vi "SteppperMotorTest.vi"() -> ()   [LabVIEW 2019]
uses:
  WSCbot_V3_Toolkit.lvlibp/WSCBOTV3_Toolkit/IO/LowLevel/PulseCounter.ctl
  <vilib>/Platform/TimedLoop/XDataNode/timing_clust.ctl
  <vilib>/Platform/TimedLoop/XDataNode/nitl_modes.ctl
  <vilib>/Platform/TimedLoop/XDataNode/wakeup.ctl
  WSCbot_V3_Toolkit.lvlibp/WSCBOTV3_Toolkit/IO/LowLevel/IO_Chanel_DIO.ctl
  <vilib>/platform/TimedLoop/XDataNode/XDataNode.xnode
  WSCbot_V3_Toolkit.lvlibp
  <vilib>/Platform/TimedLoop/XDataNode/XDNodeRunTimeDep.lvlib
  WSCbot_V3_Toolkit.lvlibp/WSCBOTV3_Toolkit/MotorControl/LowLevel/ZaxisSlideSet.vi
panel:
  in  "PulseCounterChanel":T1
  in  "Refresh Button":bool
  out "PulseCount":i32
  in  "Stop":bool
  in  "positive/nagative":bool
  in  "Stop Button":bool
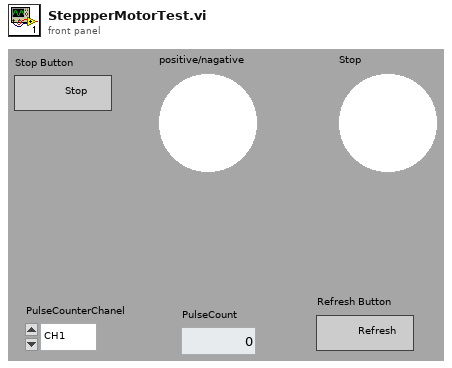
[diagram p1: front panel]
types:
  T1 = typedef "WSCbot_V3_Toolkit.lvlibp/PulseCounter.ctl" = enum16{"CH1", "CH2", "CH3", "CH4", "CH5"}
  T2 = typedef "XDNodeRunTimeDep.lvlib/timing_clust.ctl" = cluster{"Expected End [f-1]":u64, "Actual End [f-1]":u64, "Finished Late? [f-1]":bool, "Expected End [i-1]":u64, "Actual End [i-1]":u64, "Finished Late? [i-1]":bool, "Expected Start [i]":u64, "Actual Start [i]":u64, "Expected Start [f]":u64, "Actual Start [f]":u64, "Source Name":string, "Structure Name":string, "Period":i64, "Deadline":i64, "Offset":i64, "Start":i64, "Priority":i32, "Timeout":i32, "Mode":T3, "Wakeup Reason":T4, "Error":errorcluster, "Source Type":string, "Secondary Source Type":string, "Global End Time":u64, "Global Start Time":u64, "Frame Duration":u64, "Iteration Duration":u64, "Assigned CPU":i32, "I/O Scan Engine Mode":u32}
  T3 = typedef "XDNodeRunTimeDep.lvlib/nitl_modes.ctl" = enum32{"No Change", "Process missed periods, maintain original phase", "Discard missed periods, maintain original phase", "Process missed periods, ignore original phase", "Discard missed periods, ignore original phase"}
  T4 = typedef "XDNodeRunTimeDep.lvlib/wakeup.ctl" = enum32{"Normal", "Aborted", "Asynchronous wakeup", "Timing source error", "Timed loop error", "Timeout"}
  T5 = typedef "WSCbot_V3_Toolkit.lvlibp/IO_Chanel_DIO.ctl" = enum16{"A/DIO9", "A/DIO10", "C/DIO0", "C/DIO1", "C/DIO2", "C/DIO3", "C/DIO4", "C/DIO5", "C/DIO6"}
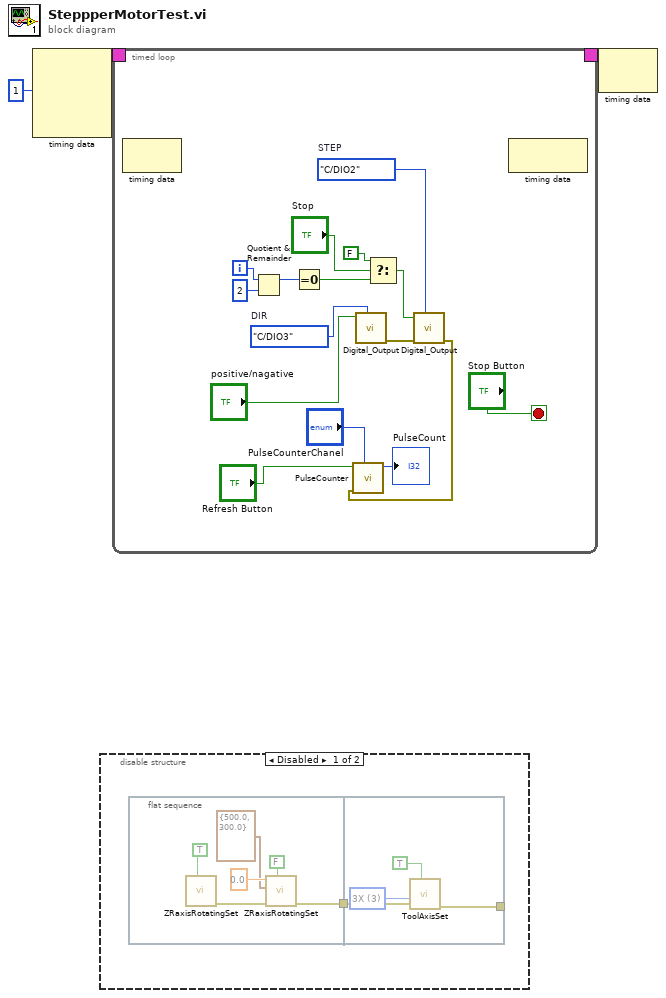
[diagram p0: block diagram]
diagram:
  n1 = node-c288(i64 1 ("Period")) -> (w3:T2)  [unwired: 3 in]
  n2 = disable-structure shown="Disabled" {
    frame Disabled {
      n3 = flat-sequence {
        tunnel: [w8] -> w4
        tunnel: w4 -> [w14]
        tunnel: [w11] -> _
        frame #0 {
          n4 = call "ZRaxisRotatingSet.vi"("Reset"=TRUE) -> ("error out"=w9:errorcluster)  [unwired: 9 in, 1 out]
          n5 = call "ZRaxisRotatingSet.vi"("Reset"=FALSE, "error in"=w9, "Velocity(deg/s)&ACC(deg/ss)"=cluster{"Velocity(cm/s)":dbl, "ACC(cm/ss)":dbl} {"Velocity(cm/s)"=500.0, "ACC(cm/ss)"=300.0}, "TargetHight(deg)"=0.0) -> ("error out"=w8:errorcluster)  [unwired: 6 in, 1 out]
        }
        frame #1 {
          w12 = u16 3 items=["0X", "1X", "2X", "3X"] ("findHomeVel (times)")
          n6 = call-poly "ToolAxisSet.vi"("Reset"=TRUE, "error in"=w14, "findHomeVel (times)"=w12) -> ("error out"=w11:errorcluster)  [unwired: 7 in, 1 out]
        }
      }
    }
    frame Enabled {
    }
  }
  n7 = timed-loop {
    timing: w3 -> [_]
    timing-out: [_] -> w2
    i -> [w22]
    stop <- "Stop Button" stop-if-true
    w29 = IO_Chanel_DIO."C/DIO3"  # DIR
    w30 = IO_Chanel_DIO."C/DIO2"  # STEP
    n8 = node-c288() -> ()  [unwired: 1 in, 1 out]
    n9 = Quotient & Remainder(x=w22, y=2) -> (x-y*floor(x/y)=w20:i32)  [unwired: 1 out]
    n10 = Equal To 0?(x=w20) -> (x = 0?=w19:bool)
    n11 = call "Digital_Output.vi"("IO_Chanel"=w29, "False/True"="positive/nagative") -> ("error out"=w23:errorcluster)  [unwired: 9 in]
    n12 = Select(t=FALSE ("s"), s="Stop", f=w19) -> (s? t:f=w25:bool)
    n13 = call "Digital_Output.vi"("IO_Chanel"=w30, "error in"=w23, "False/True"=w25) -> ("error out"=w16:errorcluster)  [unwired: 8 in]
    n14 = call "PulseCounter.vi"("PulseCounterChanel"="PulseCounterChanel", "error in"=w16, "Reset"="Refresh Button") -> ("PulseCount"=→"PulseCount":i32)  [unwired: 7 in, 1 out]
    n15 = node-c288() -> ()  [unwired: 1 in, 1 out]
  }
  n16 = node-c288(w2) -> ()  [unwired: 1 out]
